vi "LeadScrewAuto.vi"(8 "error in (no error)":errorcluster, 11 "LeadScrew":dbl) -> (0 "error out":errorcluster)   [LabVIEW 2012]
uses:
  Robot Global Data.vi
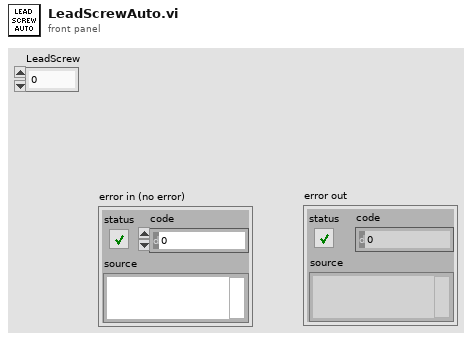
[diagram p1: front panel]
types:
  T1 = cluster{"Shoot":bool, "Enable_Targeting":bool, "Shooter":dbl, "LeadScrew":dbl, "Feed":bool, "Pickup":bool, "LiftHooks":bool, "Vision On":bool, "Vision Off":bool, "DownHooks":bool}
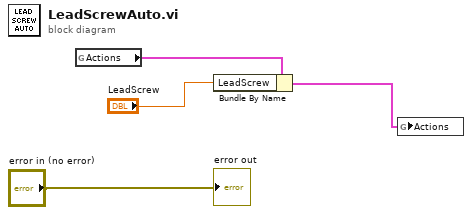
[diagram p0: block diagram]
diagram:
  n1 = global read "Robot Global Data.vi" "Actions"() -> (w4:T1)
  n2 = Bundle By Name(cluster=w4, "LeadScrew"="LeadScrew") -> (w3:T1)
  n3 = global write "Robot Global Data.vi" "Actions"(w3) -> ()
  "error out" <- "error in (no error)"
